vi "Complex Generalized Eigenvalues and Vectors.vi"(6 "output option":T1=1 items=["Eigenvalues", "Eigenvalues & Vectors"], 7 "B":T2, 8 "A":T2) -> (0 "error":i32, 2 "Eigenvectors":T2, 3 "Eigenvalues":cdb[](array[numeric]) format="%.2f")   [LabVIEW 2014, in "NI_AALPro.lvlib"]
doc: "Computes the generalized right eigenvalues and eigenvectors of the matrix pair <B>A</B> and <B>B</B>. The data types you wire to the <B>A</B> and <B>B</B> inputs determine the polymorphic instance to use."
uses:
  NI_AALPro.lvlib
  ComplexMatrix.ctl
  Eigenvalue and Vectors Output Option.ctl
  lvanlys.dll
  NI_Matrix.lvlib
panel:
  # "Complex Generalized Eigenvalues and Vectors"
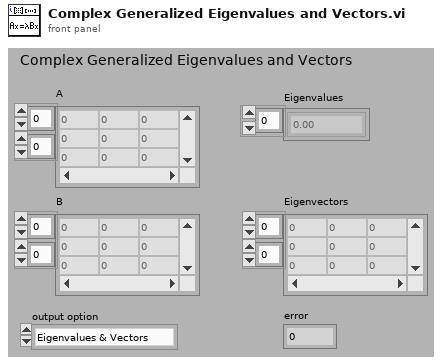
[diagram p1: front panel]
types:
  T1 = typedef "NI_AALPro.lvlib/Eigenvalue and Vectors Output Option.ctl" = i32
  T2 = typedef "NI_Matrix.lvlib/ComplexMatrix.ctl" = cdb[][]
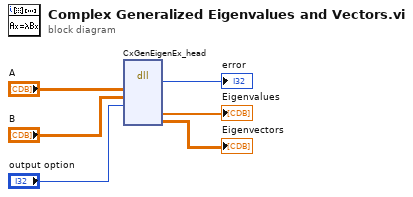
[diagram p0: block diagram]
diagram:
  n1 = dll-call lib="C:/Program Files (x86)/National Instruments/LabVIEW 2014/resource/lvanlys.*" fn="CxGenEigenEx_head"("A"="A", "B"="B", "otype"="output option") -> (→"error":i32, "Eigenvalues"=→"Eigenvalues":cdb[], "Eigenvectors"=→"Eigenvectors":T2)  [unwired: 8 in, 2 out]
